vi "LEP_RV_CreateInfoCluster.vi"(0 "Active File Count":i32, 1 "TopLevelVI":path, 2 "Error Indicator":bool[](array[boolean]), 3 "Build Path":path, 4 "UV Project File":path, 5 "error IO":errorcluster, 6 "Config":T3={"Enable debugging"=FALSE, "Debug Options"=0, "Use stack variables"=FALSE, "Generate serial only"=FALSE, "Generate guard code"=FALSE, "Generate Integer Only"=FALSE, "Generate C Function Calls"=FALSE, "ExpressionFolding"=FALSE, "Constant Allocation"=0, "Constant Deallocation"=0, "Build Specification ID"="", "Preprocessor symbols (define)"="", "Compiler Flags"="", "Linker Flags"="", "Mode"=1, "Optimization"=0, "Optimize for time"=FALSE, "Enable cross-module optimization"=FALSE, "Include paths"=[], "Optimize heap size"=TRUE, "Use MicroLib"=FALSE, "Debug Mode"=2, "Enable profile information"=FALSE, "Host name"="board", "Use DHCP"=TRUE, "IP address"="", "Subnet mask"="", "Gateway"="", "Primary DNS"="0.0.0.0", "Secondary DNS"="0.0.0.0", "MAC in target memory"=TRUE, "MAC address"="", "Console output"=1, "Target serial port"=1} {"Constant Deallocation" items=["Out of Scope", "VI End", "Application End"]; "Constant Allocation" items=["First Use", "Containing Loop", "VI Initialization", "Application Initialization"]; "Target serial port" items=["0", "1", "2", "3"]; "Console output" items=["Processor status window", "Serial port"]; "Optimization" items=["Level 0 (-O0)", "Level 1 (-O1)", "Level 2 (-O2)", "Level 3 (-O3)"]; "Mode" items=["ARM-Mode", "Thumb-Mode"]; "Debug Options" items=["Use ULINK Debugger", "Use Simulator"]; "Debug Mode" items=["Instrumented (serial port)", "Instrumented (TCP/IP)", "Non-instrumented (JTAG/USB)"]}, 7 "Target Name":string, 8 "error string":string, 9 "Message List":string[][](array[string]), 11 "File List":path[](array[path]), 12 "Node ID List":i32[](array[numeric]), 13 "Commands":T1, 19 "action":T2) -> (14 "output cluster":refnum<vi>, 15 "occurrence":refnum<k4>, 18 "error out":errorcluster)   [LabVIEW 2011]
uses:
  LEP_RV_Commands.ctl
  <vilib>/Platform/EmbProject/utilities/Emb_Utility_AppAction.ctl
  LEP_RV_Config.ctl
  <vilib>/Platform/EmbProject/Plugins/utilities/LEP_Utilities_GetSetProjectData_U32.vi
  <vilib>/Platform/EmbProject/Plugins/utilities/LEP_Utilities_GetSetProjectData_String.vi
panel:
  out "output cluster":T4 {"Config"."Constant Deallocation" items=["Out of Scope", "VI End", "Application End"]; "Config"."Constant Allocation" items=["First Use", "Containing Loop", "VI Initialization", "Application Initialization"]; "Config"."Target serial port" items=["0", "1", "2", "3"]; "Config"."Console output" items=["Processor status window", "Serial port"]; "Config"."Optimization" items=["Level 0 (-O0)", "Level 1 (-O1)", "Level 2 (-O2)", "Level 3 (-O3)"]; "Config"."Mode" items=["ARM-Mode", "Thumb-Mode"]; "Config"."Debug Options" items=["Use ULINK Debugger", "Use Simulator"]; "Config"."Debug Mode" items=["Instrumented (serial port)", "Instrumented (TCP/IP)", "Non-instrumented (JTAG/USB)"]}
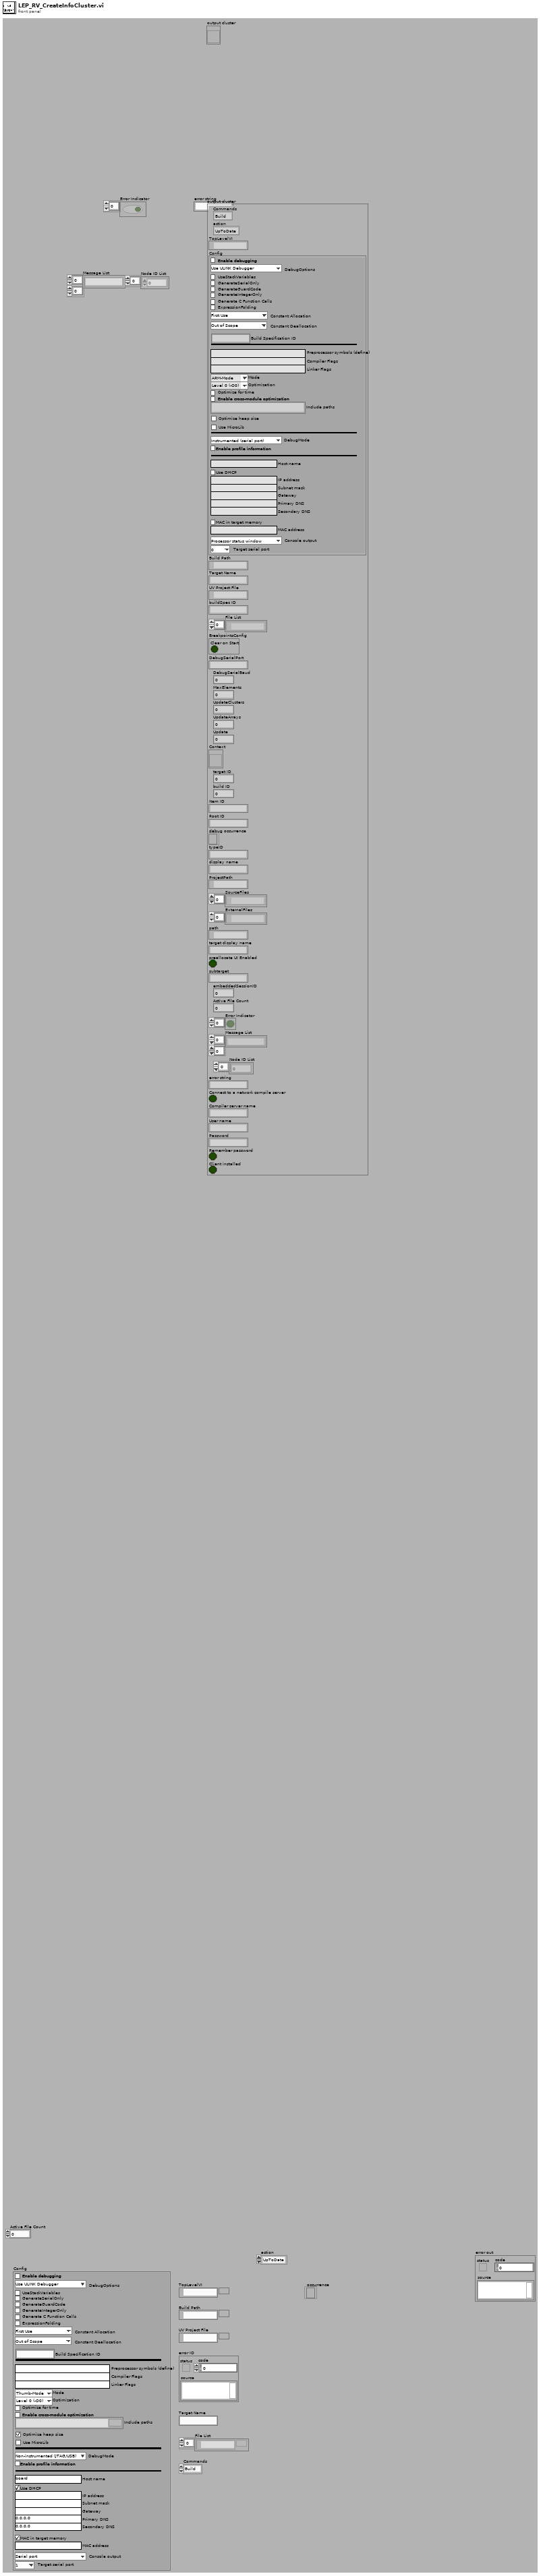
[diagram p1: front panel]
types:
  T1 = typedef "LEP_RV_Commands.ctl" = enum16{"Build", "Rebuild", "Run", "Debug", "Profile"}
  T2 = typedef "Emb_Utility_AppAction.ctl" = enum16{"UpToDate", "Build", "Cancel", "Error"}
  T3 = typedef "LEP_RV_Config.ctl" = cluster{"Enable debugging":bool, "Debug Options":u16, "Use stack variables":bool, "Generate serial only":bool, "Generate guard code":bool, "Generate Integer Only":bool, "Generate C Function Calls":bool, "ExpressionFolding":bool, "Constant Allocation":u16, "Constant Deallocation":u16, "Build Specification ID":string, "Preprocessor symbols (define)":string, "Compiler Flags":string, "Linker Flags":string, "Mode":u16, "Optimization":u16, "Optimize for time":bool, "Enable cross-module optimization":bool, "Include paths":path[], "Optimize heap size":bool, "Use MicroLib":bool, "Debug Mode":u16, "Enable profile information":bool, "Host name":string, "Use DHCP":bool, "IP address":string, "Subnet mask":string, "Gateway":string, "Primary DNS":string, "Secondary DNS":string, "MAC in target memory":bool, "MAC address":string, "Console output":u16, "Target serial port":u16}
  T4 = cluster{"Commands":T1, "action":T2, "TopLevelVI":path, "Config":T3, "Build Path":path, "Target Name":string, "UV Project File":path, "buildSpec ID":string, "File List":path[], "BreakpointsConfig":cluster{"Clear on Start":bool}, "DebugSerialPort":string, "DebugSerialBaud":u32, "MaxElements":u32, "UpdateClusters":u32, "UpdateArrays":u32, "Update":u32, "Context":refnum<vi>, "target ID":u32, "build ID":u32, "Item ID":string, "Root ID":string, "debug occurrence":refnum<k4>, "typeID":string, "display name":string, "ProjectPath":path, "SourceFiles":path[], "ExternalFiles":path[], "path":path, "target display name":string, "preallocate UI Enabled":bool, "subtarget":string, "embeddedSessionID":u32, "Active File Count":i32, "Error Indicator":bool[], "Message List":string[][], "Node ID List":i32[], "error string":string, "Connect to a network compile server":bool, "Compiler server name":string, "User name":string, "Password":string, "Remember password":bool, "Client installed":bool}
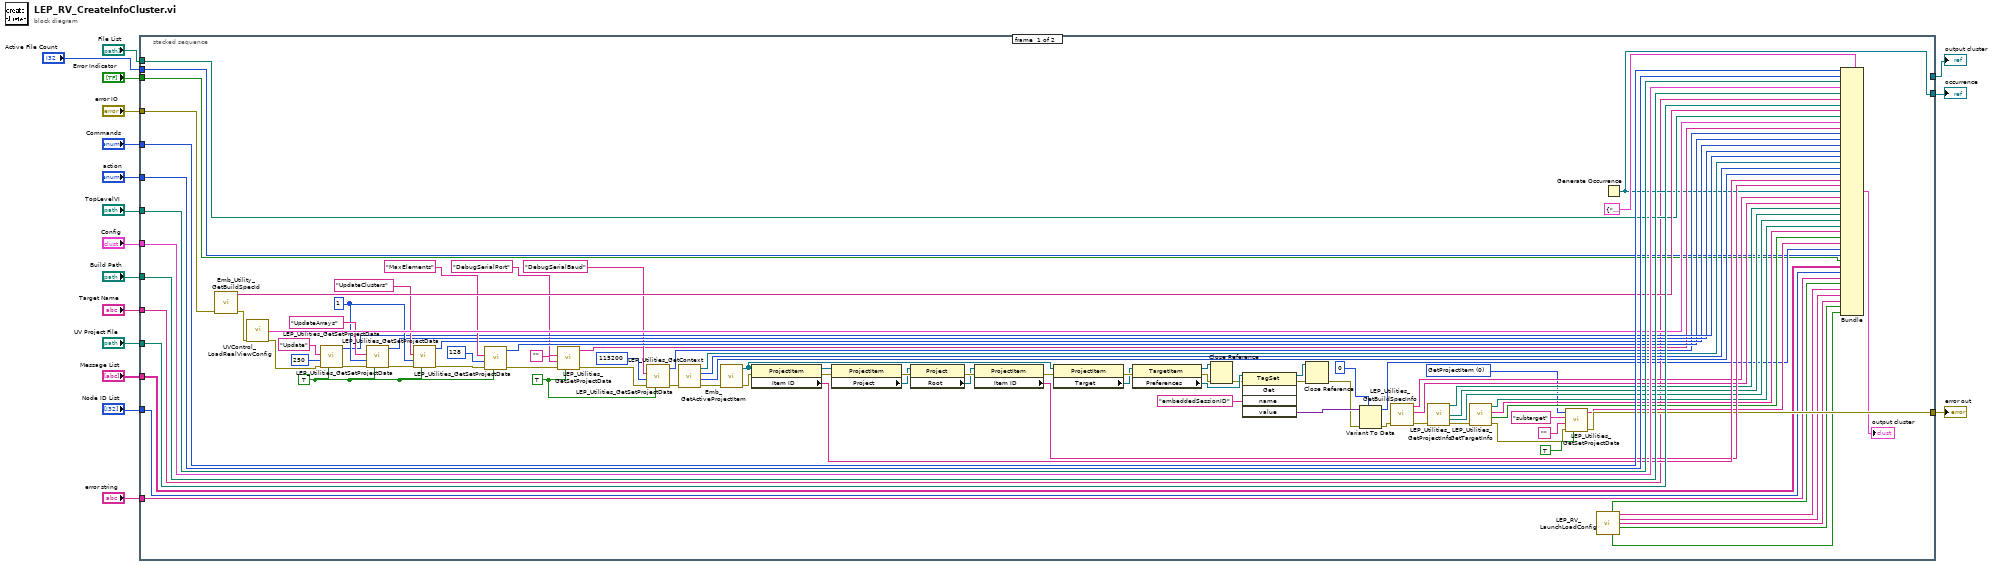
[diagram p0: block diagram]
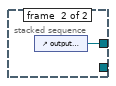
[diagram p2: hidden frame]
diagram:
  n1 = stacked-sequence {
    tunnel: "TopLevelVI" -> [w115 _]
    tunnel: "Config" -> [w114 _]
    tunnel: "Build Path" -> [w113 _]
    tunnel: "Target Name" -> [w46 _]
    tunnel: "UV Project File" -> [w112 _]
    tunnel: "action" -> [w111 _]
    tunnel: "Commands" -> [w110 _]
    tunnel: "error IO" -> [w108 _]
    tunnel: "File List" -> [w107 _]
    tunnel: [w48 _] -> w16
    tunnel: [w64 _] -> w17
    tunnel: "Active File Count" -> [w29 _]
    tunnel: "Error Indicator" -> [w27 _]
    tunnel: "Message List" -> [w26 _]
    tunnel: "Node ID List" -> [w25 _]
    tunnel: "error string" -> [w28 _]
    tunnel: [_ w116] -> w1
    frame #0 {
      w50 = u16 0 items=["GetProjectItem", "SetProjectItem"] ("Command")
      w83 = TRUE ("access target data (F)")
      w94 = TRUE ("access target data (F)")
      w99 = u32 1
      n2 = call <vilib>:"Emb_Utility_GetBuildSpecId.vi"("error in (no error)"=w108) -> ("error out"=w106:errorcluster, "buildSpec ID"=w109:string)  [unwired: 7 out]
      n3 = call "UVControl_LoadRealViewConfig.vi"("error in (no error)"=w106) -> ("BreakpointsConfig"=w105:cluster{"Clear on Start":bool}, "error out"=w93:errorcluster)  [unwired: 13 out]
      n4 = call-poly <vilib>:"LEP_Utilities_GetSetProjectData.vi"("access target data (F)"=w94, "error in"=w93, "data in"=u32 250, "ItemName"="Update") -> ("error out"=w102:errorcluster, "data out"=w91:u32)  [unwired: 1 in, 5 out]
      n5 = call-poly <vilib>:"LEP_Utilities_GetSetProjectData.vi"("access target data (F)"=w94, "error in"=w102, "data in"=w99, "ItemName"="UpdateArrays") -> ("error out"=w98:errorcluster, "data out"=w90:u32)  [unwired: 1 in, 5 out]
      n6 = call-poly <vilib>:"LEP_Utilities_GetSetProjectData.vi"("access target data (F)"=w94, "error in"=w98, "data in"=w99, "ItemName"="UpdateClusters") -> ("error out"=w97:errorcluster, "data out"=w89:u32)  [unwired: 1 in, 5 out]
      n7 = call-poly <vilib>:"LEP_Utilities_GetSetProjectData.vi"("access target data (F)"=w94, "error in"=w97, "data in"=u32 128, "ItemName"="MaxElements") -> ("error out"=w81:errorcluster, "data out"=w88:u32)  [unwired: 1 in, 5 out]
      n8 = call-poly <vilib>:"LEP_Utilities_GetSetProjectData.vi"("access target data (F)"=w83, "error in"=w81, "data in"="", "ItemName"="DebugSerialPort" ("Name")) -> ("error out"=w84:errorcluster, "data out"=w80:string)  [unwired: 1 in, 5 out]
      n9 = call-poly <vilib>:"LEP_Utilities_GetSetProjectData.vi"("access target data (F)"=w83, "error in"=w84, "data in"=u32 115200, "ItemName"="DebugSerialBaud") -> ("error out"=w78:errorcluster, "data out"=w79:u32)  [unwired: 1 in, 5 out]
      n10 = call <vilib>:"LEP_Utilities_GetContext.vi"("error in"=w78) -> ("error out"=w65:errorcluster, "build ID"=w68:u32, "target ID"=w69:u32, "Context"=w77:refnum<vi>)  [unwired: 7 out]
      n11 = call "Emb_GetActiveProjectItem.vi"("error in (no error)"=w65) -> ("error out"=w76:errorcluster, "ProjectItem Refnum"=w33:refnum<vi>)  [unwired: 9 out]
      n12 = property class="ProjectItem"(reference=w33, error in=w76) -> (reference out=w74:refnum<vi>, error out=w75:errorcluster, "Item ID"=w67:string)
      n13 = property class="ProjectItem"(reference=w74, error in=w75) -> (error out=w73:errorcluster, "Project"=w72:refnum<vi>)  [unwired: 1 out]
      n14 = property class="Project"(reference=w72, error in=w73) -> (error out=w71:errorcluster, "Root"=w70:refnum<vi>)  [unwired: 1 out]
      n15 = property class="ProjectItem"(reference=w70, error in=w71) -> (error out=w32:errorcluster, "Item ID"=w66:string)  [unwired: 1 out]
      n16 = property class="ProjectItem"(reference=w33, error in=w32) -> (error out=w40:errorcluster, "Target"=w39:refnum<vi>)  [unwired: 1 out]
      n17 = property class="TargetItem"(reference=w39, error in=w40) -> (reference out=w35:refnum<vi>, error out=w44:errorcluster, "Preferences"=w45:refnum<vi>)
      n18 = Close Reference(reference=w35, error in (no error)=w44) -> (error out=w36:errorcluster)
      n19 = invoke class="TagSet" method="Get"(reference=w45, error in=w36, "name"="embeddedSessionID" ("Name")) -> (reference out=w37:refnum<vi>, error out=w38:errorcluster, "value"=w42:variant)  [unwired: 2 in, 2 out]
      n20 = Close Reference(reference=w37, error in (no error)=w38) -> (error out=w34:errorcluster)
      n21 = Variant To Data(error in=w34, type=u32 0, Variant=w42) -> (data=w30:u32, error out=w31:errorcluster)
      n22 = call <vilib>:"LEP_Utilities_GetBuildSpecInfo.vi"("error in"=w31) -> ("error out"=w63:errorcluster, "display name"=w61:string, "typeID"=w60:string)  [unwired: 8 in]
      n23 = call <vilib>:"LEP_Utilities_GetProjectInfo.vi"("error in"=w63) -> ("ProjectPath"=w59:path, "SourceFiles"=w58:path[], "ExternalFiles"=w57:path[], "error out"=w62:errorcluster)  [unwired: 10 in, 1 out]
      n24 = call <vilib>:"LEP_Utilities_GetTargetInfo.vi"("error in"=w62) -> ("error out"=w49:errorcluster, "preallocate UI Enabled"=w54:bool, "display name"=w55:string, "path"=w56:path)  [unwired: 7 in]
      n25 = call-poly <vilib>:"LEP_Utilities_GetSetProjectData.vi"("access target data (F)"=TRUE, "error in"=w49, "data in"="", "ItemName"="subtarget", "Command"=w50) -> ("error out"=w48:errorcluster, "data out"=w47:string)  [unwired: 4 in, 1 out]
      n26 = call "LEP_RV_LaunchLoadConfig.vi"() -> ("Connect to a network compile server"=w19:bool, "Compiler server name"=w20:string, "User name"=w21:string, "Password"=w22:string, "Remember password"=w23:bool, "Client installed"=w24:bool)  [unwired: 8 in, 2 out]
      n27 = Generate Occurrence() -> (w64:refnum<k4>)
      n28 = Bundle(cluster=T4 {"Commands"=enum."Build", "action"=enum."UpToDate", "TopLevelVI"=path "", "Config"={"Enable debugging"=FALSE, "Debug Options"=0, "Use stack variables"=FALSE, "Generate serial only"=FALSE, "Generate guard code"=FALSE, "Generate Integer Only"=FALSE, "Generate C Function Calls"=FALSE, "ExpressionFolding"=FALSE, "Constant Allocation"=0, "Constant Deallocation"=0, "Build Specification ID"="", "Preprocessor symbols (define)"="", "Compiler Flags"="", "Linker Flags"="", "Mode"=0, "Optimization"=0, "Optimize for time"=FALSE, "Enable cross-module optimization"=FALSE, "Include paths"=[], "Optimize heap size"=FALSE, "Use MicroLib"=FALSE, "Debug Mode"=0, "Enable profile information"=FALSE, "Host name"="", "Use DHCP"=FALSE, "IP address"="", "Subnet mask"="", "Gateway"="", "Primary DNS"="", "Secondary DNS"="", "MAC in target memory"=FALSE, "MAC address"="", "Console output"=0, "Target serial port"=0}, "Build Path"=path "", "Target Name"="", "UV Project File"=path "", "buildSpec ID"="", "File List"=[], "BreakpointsConfig"={"Clear on Start"=FALSE}, "DebugSerialPort"="", "DebugSerialBaud"=0, "MaxElements"=0, "UpdateClusters"=0, "UpdateArrays"=0, "Update"=0, "Context"=refnum, "target ID"=0, "build ID"=0, "Item ID"="", "Root ID"="", "debug occurrence"=refnum, "typeID"="", "display name"="", "ProjectPath"=path "", "SourceFiles"=[], "ExternalFiles"=[], "path"=path "", "target display name"="", "preallocate UI Enabled"=FALSE, "subtarget"="", "embeddedSessionID"=0, "Active File Count"=0, "Error Indicator"=[], "Message List"=[], "Node ID List"=[], "error string"="", "Connect to a network compile server"=FALSE, "Compiler server name"="", "User name"="", "Password"="", "Remember password"=FALSE, "Client installed"=FALSE} ("output cluster"), "Commands"=w110, "action"=w111, "TopLevelVI"=w115, "Config"=w114, "Build Path"=w113, "Target Name"=w46, "UV Project File"=w112, "buildSpec ID"=w109, "File List"=w107, "BreakpointsConfig"=w105, "DebugSerialPort"=w80, "DebugSerialBaud"=w79, "MaxElements"=w88, "UpdateClusters"=w89, "UpdateArrays"=w90, "Update"=w91, "Context"=w77, "target ID"=w69, "build ID"=w68, "Item ID"=w67, "Root ID"=w66, "debug occurrence"=w64, "typeID"=w60, "display name"=w61, "ProjectPath"=w59, "SourceFiles"=w58, "ExternalFiles"=w57, "path"=w56, "target display name"=w55, "preallocate UI Enabled"=w54, "subtarget"=w47, "embeddedSessionID"=w30, "Active File Count"=w29, "Error Indicator"=w27, "Message List"=w26, "Node ID List"=w25, "error string"=w28, "Connect to a network compile server"=w19, "Compiler server name"=w20, "User name"=w21, "Password"=w22, "Remember password"=w23, "Client installed"=w24) -> (→"output cluster":T4)
    }
    frame #1 {
      n29 = control-ref of="output cluster"() -> (w116:refnum<vi>)
    }
  }
  "occurrence" <- w17
  "error out" <- w16
  "output cluster" <- w1
